vi "GLIMPSE frame skip test.vi"(4 "error in (no error)":errorcluster) -> (0 "error out":errorcluster)   [LabVIEW 2011]
uses:
  GLIMPSE Globals.vi
  <vilib>/vision/NI_Vision_Development_Module.lvlib
  <vilib>/Analysis/NI_AALPro.lvlib
panel:
  out "Histogram":T1(graph)
  in  "Time delay (ms)":u32=1000
  out "Delta angle":dbl(graph)
  in  "Input from existing":path=path "d:/1.glimpse"
  out "Progress":i16(slide) scale=0.0..1240.0
  in  "Quit":bool
  in  "Go ahead":bool
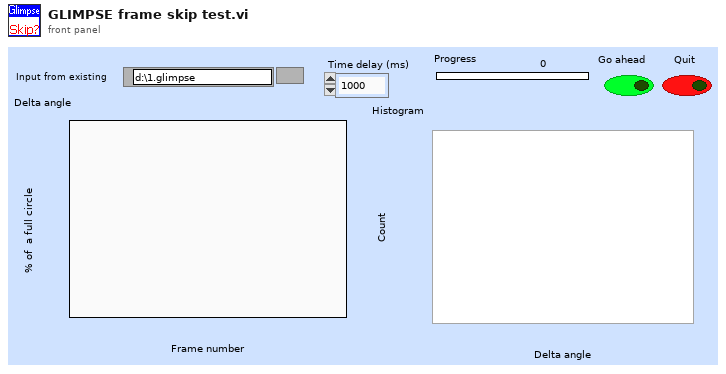
[diagram p1: front panel]
types:
  T1 = cluster{"X Values":dbl[], "Histogram: h(x)":i32[]}
  T2 = typedef "Header file data.ctl" = cluster{"Frames Acquired":u32, "Region width":i32, "Region height":i32, "Element 0 of TTB":u32, "time of 1st frame, \nsec since 1/1/04":dbl, "TTB Array (ms)":u32[], "Offsets Array":T3, "Pixel depth":u32}
  T3 = typedef "Offset table.ctl" = cluster{"offset":T4, "file number":T5}[]
  T4 = typedef "Offset.ctl" = i32
  T5 = typedef "file number.ctl" = u8
  T6 = typedef "IMAQ Image.ctl" = refnum<image>
  T7 = cluster{"Coordinates[0]":i32, "Coordinates[1]":i32, "Coordinates[2]":i32, "Coordinates[3]":i32, "Coordinates[4]":i32, "Coordinates[5]":i32, "Coordinates[6]":i32, "Coordinates[7]":i32, "Coordinates[8]":i32}
  T8 = cluster{"Coordinates[0]":i32, "Coordinates[1]":i32}
  T9 = cluster{"Left":i32, "Top":i32, "Right":i32, "Bottom":i32}
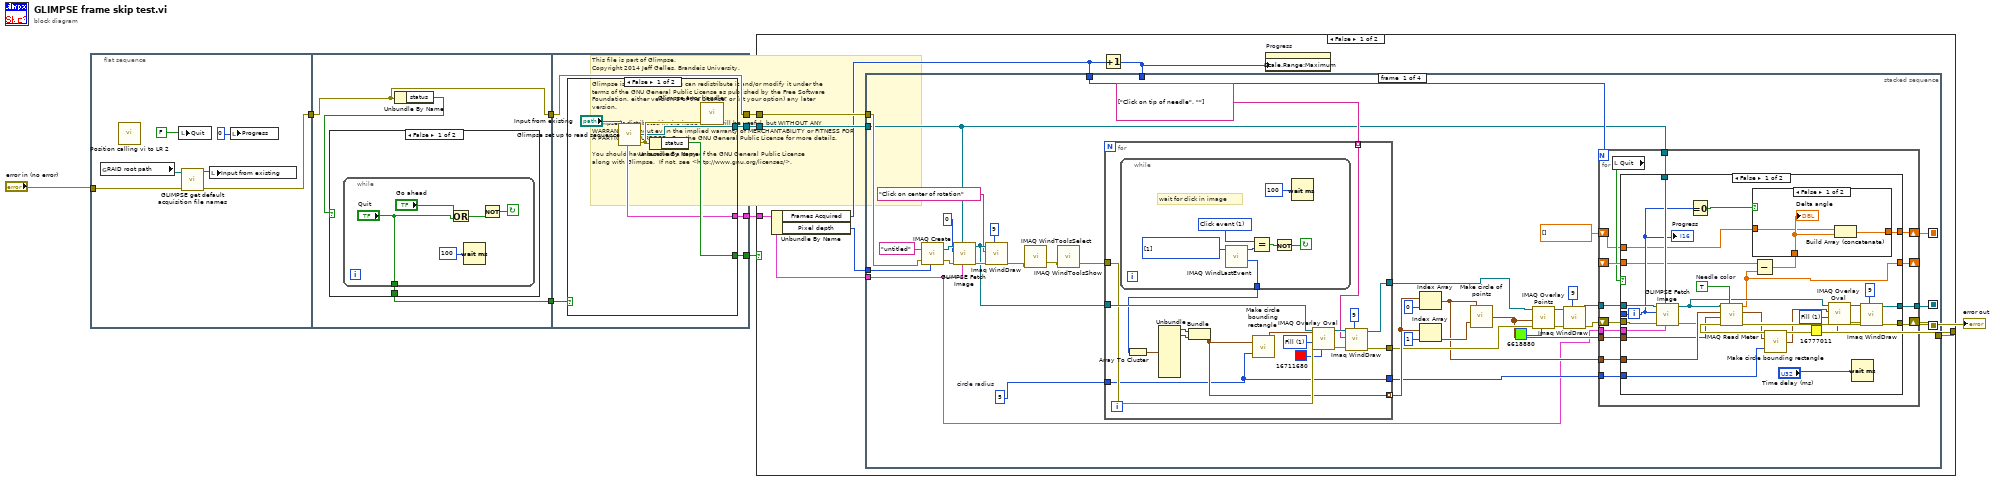
[diagram p0: block diagram]
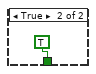
[diagram p2: hidden frame]
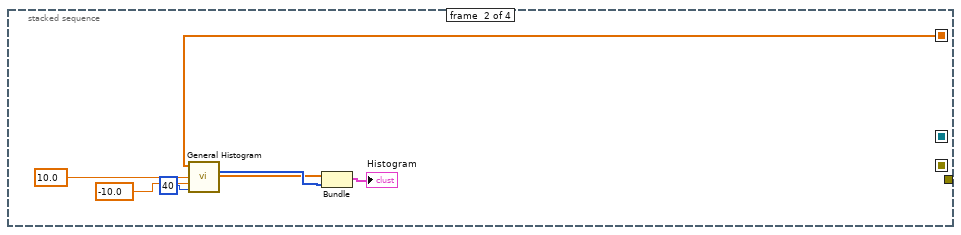
[diagram p6: hidden frame]
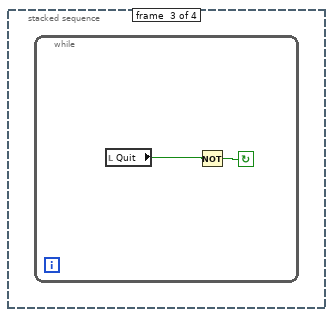
[diagram p7: hidden frame]
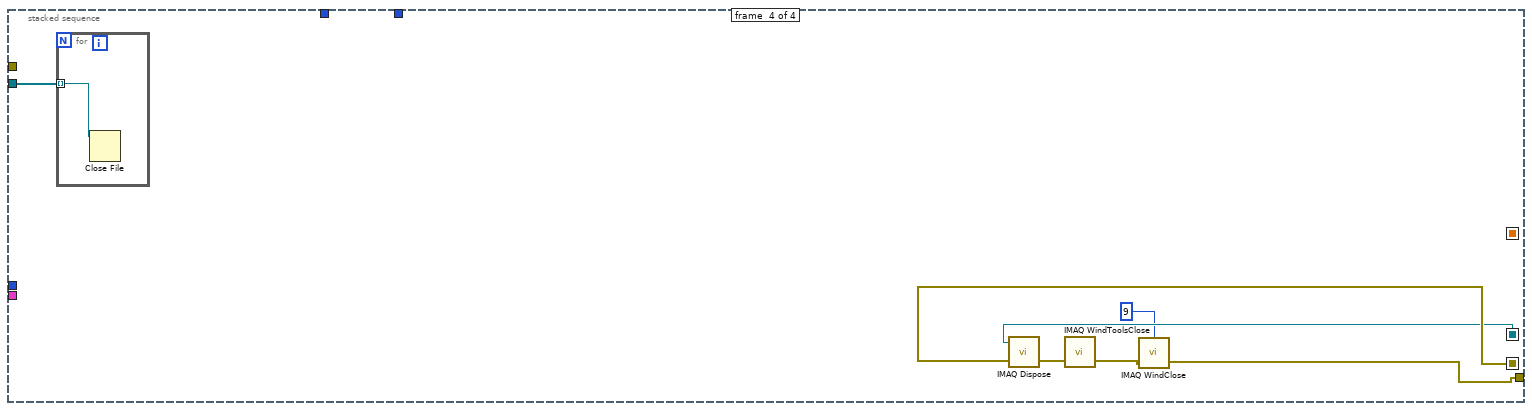
[diagram p8: hidden frame]
diagram:
  # "This file is part of Glimpse. \nCopyright 2014 Jeff Gelles, Brandeis University.    \n\nGlimpse is free software: you can redistribute it and/or modify it under the \nterms of the GNU General Public License as published by the Free Software \nFoundation, either version 3 of the License, or (at your option) any later \nversion.\n\nGlimpse is distributed in the hope that it will be useful, but WITHOUT ANY \nWARRANTY; without even the implied warranty of MERCHANTABILITY or FITNESS FOR \nA PARTICULAR PURPOSE.  See the GNU General Public License for more details.\n\nYou should have received a copy of the GNU General Public License\nalong with Glimpse.  If not, see <http://www.gnu.org/licenses/>."
  n1 = flat-sequence {
    tunnel: "error in (no error)" -> [w13]
    tunnel: [w11] -> w4
    tunnel: w4 -> [w18]
    tunnel: [w18] -> w3
    tunnel: [w16] -> w2
    tunnel: [w29] -> w8
    tunnel: [w28] -> w7
    tunnel: [w27] -> w5
    tunnel: w3 -> [w27]
    tunnel: w2 -> [w30]
    tunnel: [w26] -> w1
    frame #0 {
      n2 = global read "GLIMPSE Globals.vi" "RAID root path"() -> (w14:path)
      n3 = call "Position calling vi to LR 2.vi"() -> ()  [unwired: 2 in, 4 out]
      n4 = local write "Quit"(FALSE ("Abort")) -> ()
      n5 = call "GLIMPSE get default acquisition file names.vi"("error in"=w13, "RAID root path"=w14) -> ("error out"=w11:errorcluster, "last directory path"=w12:path)  [unwired: 6 out]
      n6 = local write "Input from existing"(w12) -> ()
      n7 = local write "Progress"(i16 0 ("Progress")) -> ()
    }
    frame #1 {
      n8 = Unbundle By Name(w18) -> ("status"=w17:bool)
      n9 = case shown="False" w17 {
        tunnel: [w19 TRUE ("Abort")] -> w16
        frame False {
          n10 = while {
            tunnel: ["Quit"] -> w19
            stop <- w24 continue-if-true
            n11 = Or(x="Go ahead", y="Quit") -> (x .or. y?=w22:bool)
            n12 = Wait (ms)(milliseconds to wait=u32 100) -> ()  [unwired: 1 out]
            n13 = Not(x=w22) -> (.not. x?=w24:bool)
          }
        }
        frame True {
        }
      }
    }
    frame #2 {
      n14 = case shown="False" w30 {
        selector: w30 -> [_ w36]
        tunnel: [w32 w36] -> w29
        tunnel: [w33 _] -> w28
        tunnel: [w31 _] -> w26
        frame False {
          n15 = call "Glimpse set up to read sequence.vi"("acquisition directory path"="Input from existing") -> ("Header file data out"=w31:T2, "Acquisition refnum array"=w33:refnum<file>[], "error out"=w34:errorcluster)  [unwired: 1 in, 3 out]
          n16 = Unbundle By Name(w34) -> ("status"=w32:bool)
          n17 = call "Glimpse error handler.vi"("error in"=w34) -> ()  [unwired: 1 in, 6 out]
        }
        frame True {
        }
      }
    }
  }
  n18 = case shown="False" w8 {
    tunnel: w7 -> [w43 _]
    tunnel: [w40 w173] -> w6
    tunnel: w5 -> [w41 w173]
    tunnel: w1 -> [w37 _]
    frame False {
      n19 = Unbundle By Name(w37) -> ("Frames Acquired"=w39:u32, "Pixel depth"=w38:u32)
      n20 = Increment(x=w39) -> (x+1=w42:u32)
      n21 = stacked-sequence {
        seq-local: [w50 _ _ _] -> [_ _ _ w170]
        seq-local: [w49 _ _ _] -> [_ _ _ w166]
        seq-local: [w46 _ _ _] -> [_ w161 _ _]
        tunnel: w43 -> [w48 _ _ w171]
        tunnel: w42 -> [_ _ _ _]
        tunnel: w39 -> [w53 _ _ _]
        tunnel: w41 -> [w52 _ _ _]
        tunnel: [_ _ _ w167] -> w40
        tunnel: w38 -> [w45 _ _ _]
        tunnel: w37 -> [w44 _ _ _]
        frame #0 {
          w75 = 5  # circle radius
          n22 = call "IMAQ Create"("Image Name"="untitled", "Image Type"=w45, "error in (no error)"=w52) -> ("New Image"=w80:T6, "error out"=w79:errorcluster)  [unwired: 1 in, 1 out]
          n23 = call "GLIMPSE Fetch Image.vi"("Header file data"=w44, "Acqisition files refnums"=w48, "error in"=w79, "Logical Frame Number\n(starting with zero)"=0 ("Logical Frame Number\n(starting with zero)"), "Image In"=w80) -> ("error out"=w78:errorcluster, "Image Out"=w74:T6)  [unwired: 2 in, 3 out]
          n24 = call "Imaq WindDraw"("Window Number (0...15)"=9, "error in (no error)"=w78, "Title"="Click on center of rotation", "Image"=w74) -> ("error out"=w71:errorcluster)  [unwired: 2 in, 5 out]
          n25 = call "IMAQ WindToolsSelect"("error in (no error)"=w71) -> ("error out"=w70:errorcluster)  [unwired: 3 in, 2 out]
          n26 = call "IMAQ WindToolsShow"("error in (no error)"=w70) -> ("error out"=w76:errorcluster)  [unwired: 2 in, 3 out]
          n27 = for {
            tunnel: w75 -> [w132]
            tunnel: w74 -> [w148]
            tunnel: w76 -> [w147]
            tunnel: string[] ["Click on tip of needle", ""] -> [w140] mode=indexing
            tunnel: [w133] -> w66 mode=indexing
            tunnel: [w138] -> w65
            tunnel: [w135] -> w60
            tunnel: [w132] -> w55
            w145 = u32 1 items=["Frame", "Fill"] ("Drawing Mode (Frame)")
            n28 = while {
              tunnel: [w150] -> w139
              stop <- w151 continue-if-true
              w153 = 1 items=["No  event", "Click event", "Draw event", "Move event", "Size event", "Scroll event", "Activate event", "Close event", "Double click event"]
              w155 = i32[] [1] items=["No  event", "Click event", "Draw event", "Move event", "Size event", "Scroll event", "Activate event", "Close event", "Double click event"] ("Events list (all)")
              # "wait for click in image"
              n29 = call "IMAQ WindLastEvent"("Events list (all)"=w155) -> ("Coordinates"=w150:i32[], "Event"=w154:i32)  [unwired: 1 in, 8 out]
              n30 = Equal?(x=w153, y=w154) -> (x = y?=w152:bool)
              n31 = Not(x=w152) -> (.not. x?=w151:bool)
              n32 = Wait (ms)(milliseconds to wait=u32 100) -> ()  [unwired: 1 out]
            }
            n33 = Array To Cluster(array=w139) -> (cluster=w134:T7)
            n34 = Unbundle(w134) -> ("Coordinates[0]"=w137:i32, "Coordinates[1]"=w136:i32)  [unwired: 7 out]
            n35 = Bundle("Coordinates[0]"=w137, "Coordinates[1]"=w136) -> (w133:T8)  [unwired: 1 out]
            n36 = call "Make circle bounding rectangle.vi"("circle radius"=w132, "Coordinates"=w133) -> ("Bounding Rectangle"=w146:T9)
            n37 = call "IMAQ Overlay Oval"("Color"=u32 16711680, "error in (no error)"=w147, "Drawing Mode (Frame)"=w145, "Bounding Rectangle"=w146, "Image"=w148) -> ("error out"=w142:errorcluster, "Image Out"=w141:T6)  [unwired: 1 in, 4 out]
            n38 = call "Imaq WindDraw"("Window Number (0...15)"=9, "error in (no error)"=w142, "Title"=w140, "Image"=w141) -> ("error out"=w135:errorcluster, "Image Out (duplicate)"=w138:T6)  [unwired: 2 in, 4 out]
          }
          n39 = Index Array(array=w66, index=0) -> (element=w58:T8)
          n40 = Index Array(array=w66, index=1) -> (element=w61:T8)
          n41 = call "Make circle of points.vi"("Periphery"=w61, "Center"=w58) -> ("Array of Points"=w57:cluster{"X":i32, "Y":i32}[])
          n42 = call "IMAQ Overlay Points"("Color"=u32 6618880, "error in (no error)"=w60, "Array of Points"=w57, "Image"=w65) -> ("error out"=w63:errorcluster, "Image Out"=w62:T6)  [unwired: 2 in, 4 out]
          n43 = call "Imaq WindDraw"("Window Number (0...15)"=9, "error in (no error)"=w63, "Image"=w62) -> ("error out"=w51:errorcluster, "Image Out (duplicate)"=w59:T6)  [unwired: 3 in, 4 out]
          n44 = for {
            N: w53 -> [_]
            tunnel: w59 -> [w92]
            tunnel: w58 -> [w95]
            tunnel: w57 -> [w94]
            tunnel: w55 -> [w93]
            shift-right: [w91] -> w50
            shift-left: w51 -> [w90]
            tunnel: [w89] -> w49
            tunnel: w48 -> [w88]
            shift-right: [w85] -> _
            shift-left: _ -> [w86]
            shift-right: [w83] -> w46
            shift-left: dbl[] [] -> [w82]
            tunnel: w44 -> [w81]
            i -> [w87]
            n45 = local read "Quit"() -> (w84:bool)
            n46 = case shown="False" w84 {
              tunnel: w95 -> [w122 _]
              tunnel: w94 -> [w121 _]
              tunnel: w93 -> [w112 _]
              tunnel: w92 -> [w109 w130]
              tunnel: [w108 w129] -> w91
              tunnel: w90 -> [w107 w129]
              tunnel: [w106 w130] -> w89
              tunnel: w88 -> [w105 _]
              tunnel: w87 -> [w103 _]
              tunnel: w86 -> [w102 w131]
              tunnel: [w101 w131] -> w85
              tunnel: [w98 w128] -> w83
              tunnel: w82 -> [w97 w128]
              tunnel: w81 -> [w96 _]
              frame False {
                w120 = u32 1 items=["Frame", "Fill"] ("Drawing Mode (Frame)")
                w123 = TRUE  # Needle color
                n47 = call "GLIMPSE Fetch Image.vi"("Header file data"=w96, "Acqisition files refnums"=w105, "error in"=w107, "Logical Frame Number\n(starting with zero)"=w103, "Image In"=w109) -> ("error out"=w110:errorcluster, "Image Out"=w111:T6)  [unwired: 2 in, 3 out]
                n48 = Equal To 0?(x=w103) -> (x = 0?=w104:bool)
                n49 = call "IMAQ Read Meter"("Needle color"=w123, "error in (no error)"=w110, "Arc Points"=w121, "Needle Base"=w122, "Image"=w111) -> ("error out"=w115:errorcluster, "Point"=w114:cluster{"X":sgl, "Y":sgl}, "Percentage of scale"=w101:dbl)  [unwired: 4 out]
                n50 = Subtract(x=w102, y=w101) -> (x-y=w100:dbl)
                n51 = case shown="False" w104 {
                  tunnel: w100 -> [w126 _]
                  tunnel: [w125 w127] -> w98
                  tunnel: w97 -> [w124 w127]
                  frame False {
                    n52 = Build Array (concatenate)(w124, w126) -> (w125:dbl[])
                    "Delta angle" <- w126
                  }
                  frame True {
                  }
                }
                n53 = call "Make circle bounding rectangle.vi"("circle radius"=w112, "Coordinates"=w114) -> ("Bounding Rectangle"=w113:T9)
                n54 = call "IMAQ Overlay Oval"("Color"=u32 16777011, "error in (no error)"=w115, "Drawing Mode (Frame)"=w120, "Bounding Rectangle"=w113, "Image"=w111) -> ("error out"=w117:errorcluster, "Image Out"=w116:T6)  [unwired: 1 in, 4 out]
                n55 = Wait (ms)(milliseconds to wait="Time delay (ms)") -> ()  [unwired: 1 out]
                n56 = call "Imaq WindDraw"("Window Number (0...15)"=9, "error in (no error)"=w117, "Image"=w116) -> ("error out"=w108:errorcluster, "Image Out (duplicate)"=w106:T6)  [unwired: 3 in, 4 out]
                "Progress" <- w103
              }
              frame True {
              }
            }
          }
        }
        frame #1 {
          n57 = call <vilib>:"General Histogram.vi"("X"=w161, "max"=10.0, "min"=-10.0, "# bins"=40 ("intervals")) -> ("Histogram"=w159:i32[], "Axis"=w158:dbl[])  [unwired: 2 in, 8 out]
          n58 = Bundle("Axis"=w158, "Histogram"=w159) -> (→"Histogram":cluster{"Axis":dbl[], "Histogram":i32[]})  [unwired: 1 out]
        }
        frame #2 {
          n59 = while {
            stop <- w164 continue-if-true
            n60 = local read "Quit"() -> (w163:bool)
            n61 = Not(x=w163) -> (.not. x?=w164:bool)
          }
        }
        frame #3 {
          n62 = for {
            tunnel: w171 -> [w172] mode=indexing
            n63 = Close File(refnum=w172) -> ()  [unwired: 1 in, 2 out]
          }
          n64 = call "IMAQ Dispose"("Image"=w166, "error in (no error)"=w170) -> ("error out"=w169:errorcluster)  [unwired: 1 in, 3 out]
          n65 = call "IMAQ WindToolsClose"("error in (no error)"=w169) -> ("error out"=w168:errorcluster)  [unwired: 5 out]
          n66 = call "IMAQ WindClose"("Window Number (0...15)"=9, "error in (no error)"=w168) -> ("error out"=w167:errorcluster)  [unwired: 1 in, 3 out]
        }
      }
      n67 = property on="Progress" class="Slide (strict)"("Scale.Range:Maximum"=w42) -> ()  [unwired: 2 in, 2 out]
    }
    frame True {
    }
  }
  "error out" <- w6
